vi "convert color to rgb string.vi"(1 "primary":u32(colorbox)) -> (0 "String":string)   [LabVIEW 2021, in "TSC Material Theme.lvlib" / "Material-Scheme.lvclass"]
doc: "get the RGB string from the color box\n\n<b>Code Developed By:</b> +\nDaniel Coons +\nTechnology Service Corporation +\nwww.tsc.com/atcs"
uses:
  Material-Scheme.lvclass
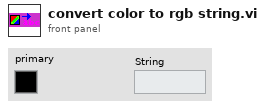
[diagram p1: front panel]
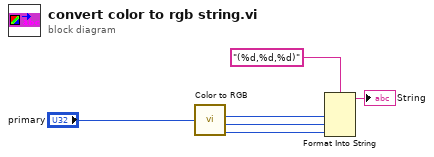
[diagram p0: block diagram]
diagram:
  n1 = call <vilib>:"Color to RGB.vi"("Color"="primary") -> ("R"=w2:u8, "G"=w3:u8, "B"=w4:u8)  [unwired: 1 out]
  n2 = Format Into String(format string="(%d,%d,%d)", w2, w3, w4) -> (resulting string=→"String":string)  [unwired: 2 in, 1 out]
